vi "dg.vi"() -> ()   [LabVIEW 2016]
panel:
  in  "?":dbl(slide) scale=0.0..150.0
  out "celsius":dbl(knob) scale=0.0..150.0
  # "farinheight"
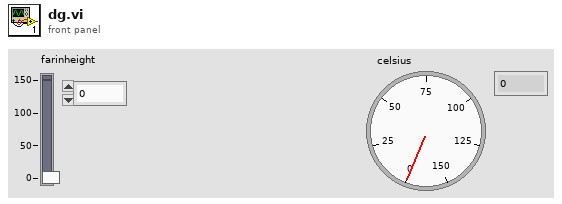
[diagram p1: front panel]
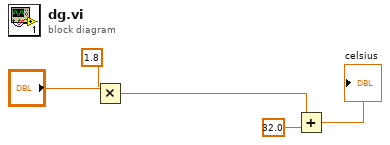
[diagram p0: block diagram]
diagram:
  n1 = Multiply(x=1.8, y="?") -> (x*y=w3:dbl)
  n2 = Add(x=w3, y=32.0) -> (x+y=→"celsius":dbl)
